vi "SQLite Gen Std.Select Statement.vi"(9 "Filter String":string, 10 "Fields":string[](array[string]), 11 "Table Name":string) -> (3 "String":string)   [LabVIEW 2021, in "EDT SQLite+.lvlib"]
uses:
  EDT SQLite+.lvlib
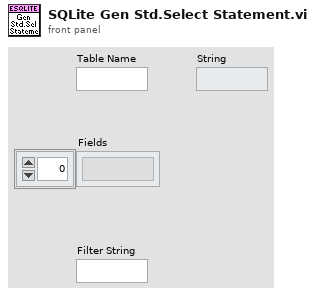
[diagram p1: front panel]
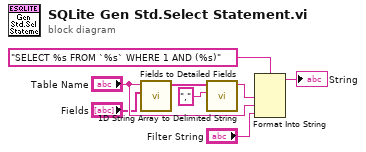
[diagram p0: block diagram]
diagram:
  n1 = call "Fields to Detailed Fields.vi"("Fields"="Fields", "Table Name"="Table Name") -> ("Detailed Fields"=w3:string[])  [unwired: 9 in]
  n2 = call <vilib>:"1D String Array to Delimited String.vi"("delimiter"=",", "string array"=w3) -> ("delimited string"=w6:string)  [unwired: 9 in]
  n3 = Format Into String(format string="SELECT %s FROM `%s` WHERE 1 AND (%s)" ("SELECT  statement"), w6, "Table Name", "Filter String") -> (resulting string=→"String":string)  [unwired: 2 in, 1 out]
